vi "HW_GEN - Data Queue Manage FGV.vi"(7 "Oper.":T3=enum."Add", 8 "error in":errorcluster, 10 "ChanTag":string, 11 "Add Chan":T2) -> (0 "error out":errorcluster, 2 "ChanInfo":cluster{"Queue Name":string, "index":i32}, 3 "AllChanInfo":T1(array[cluster]))   [LabVIEW 2016]
uses:
  Ctrls/HardWare _ Data Queue Manage FGV Operation.ctl
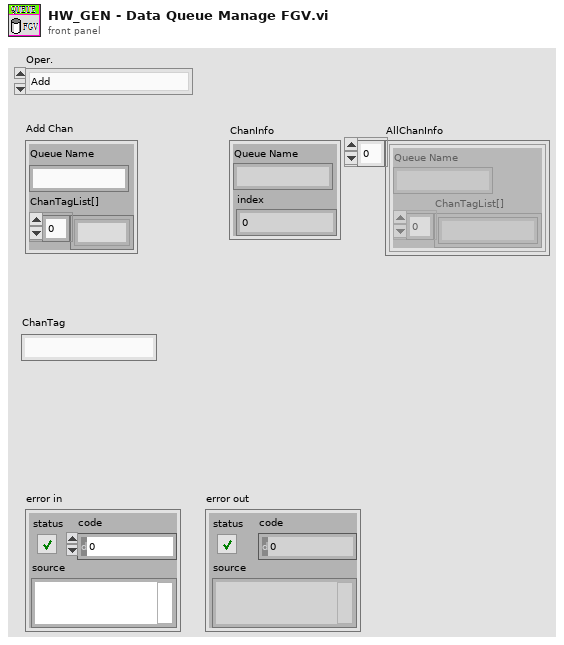
[diagram p1: front panel]
types:
  T1 = cluster{"Queue Name":string, "ChanTagList[]":string[]}[]
  T2 = cluster{"Queue Name":string, "ChanTagList[]":string[]}
  T3 = typedef "HardWare _ Data Queue Manage FGV Operation.ctl" = enum16{"Initialize", "Add", "Read", "All"}
  T4 = cluster{"Queue Name":string, "index of element":i32}
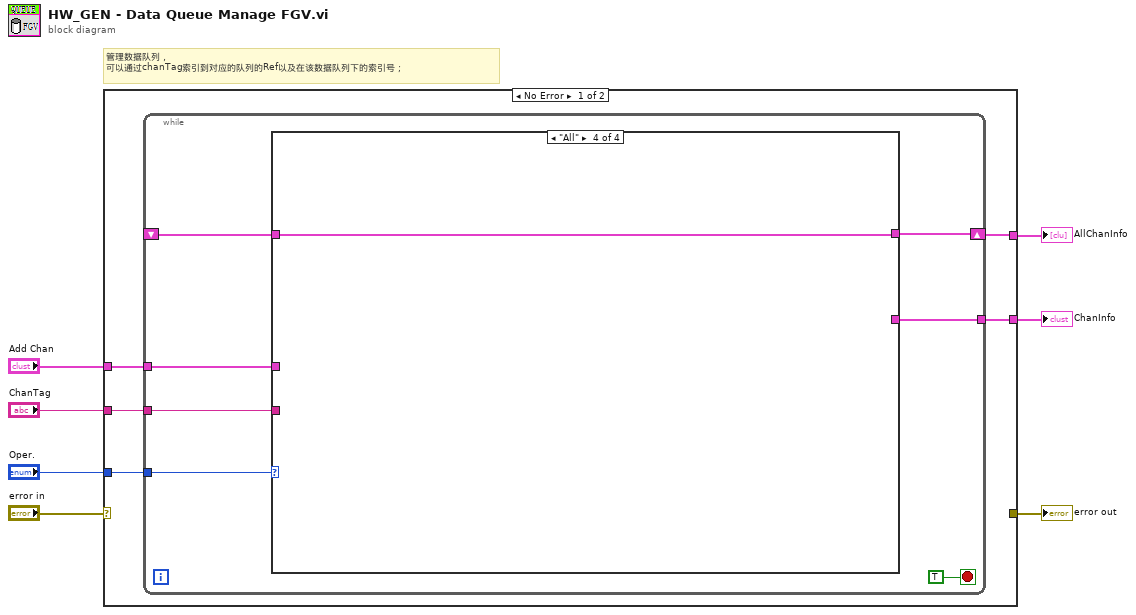
[diagram p0: block diagram]
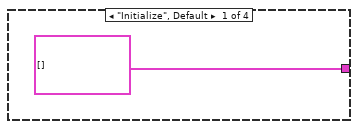
[diagram p2: hidden frame]
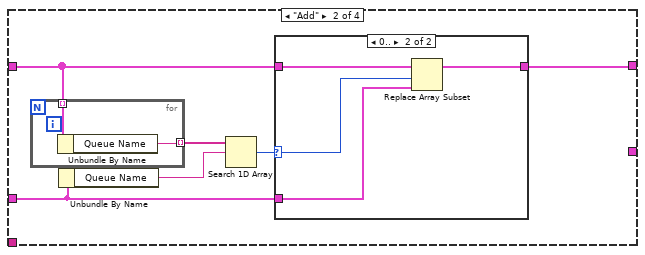
[diagram p3: hidden frame]
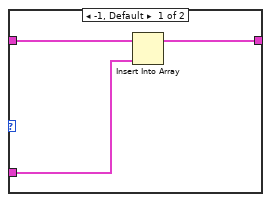
[diagram p4: hidden frame]
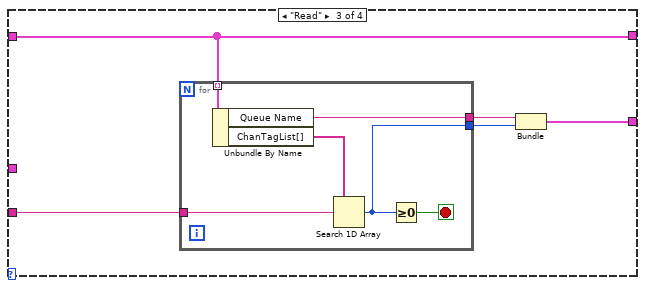
[diagram p5: hidden frame]
diagram:
  # "管理数据队列，\n可以通过chanTag索引到对应的队列的Ref以及在该数据队列下的索引号；"
  n1 = case shown="No Error" "error in" {
    selector: "error in" -> [_ w48]
    tunnel: [_ w48] -> w6
    tunnel: "Oper." -> [w12 _]
    tunnel: "Add Chan" -> [w11 _]
    tunnel: "ChanTag" -> [w10 _]
    tunnel: [w9 _] -> w2
    tunnel: [w8 _] -> w1
    frame No Error {
      n2 = while {
        tunnel: w12 -> [w18]
        tunnel: w11 -> [w17]
        tunnel: w10 -> [w16]
        shift-right: [w15] -> w8
        shift-left: _ -> [w14]
        tunnel: [w13] -> w9
        stop <- TRUE stop-if-true
        n3 = case shown="\"All\"" w18 {
          tunnel: w17 -> [_ w21 _ _]
          tunnel: w16 -> [_ _ w40 _]
          tunnel: [T1 [] w22 w39 w47] -> w15
          tunnel: w14 -> [_ w23 w39 w47]
          tunnel: [_ _ w36 _] -> w13
          frame "Initialize", Default {
          }
          frame "Add" {
            n4 = for {
              tunnel: w23 -> [w35] mode=indexing
              tunnel: [w34] -> w26 mode=indexing
              n5 = Unbundle By Name(w35) -> ("Queue Name"=w34:string)
            }
            n6 = Unbundle By Name(w21) -> ("Queue Name"=w25:string)
            n7 = Search 1D Array(1D array=w26, element=w25) -> (index of element=w24:i32)  [unwired: 1 in]
            n8 = case shown="0.." w24 {
              selector: w24 -> [_ w31]
              tunnel: w23 -> [w29 w33]
              tunnel: [w28 w32] -> w22
              tunnel: w21 -> [w27 w30]
              frame -1, Default {
                n9 = Insert Into Array(array=w29, new element=w27) -> (w28:T1)  [unwired: 1 in]
              }
              frame 0.. {
                n10 = Replace Array Subset(array=w33, new element=w30, index=w31) -> (w32:T1)
              }
            }
          }
          frame "Read" {
            n11 = for {
              tunnel: w39 -> [w46] mode=indexing
              tunnel: w40 -> [w44]
              tunnel: [w42] -> w38
              tunnel: [w41] -> w37
              stop <- w43 stop-if-true
              n12 = Unbundle By Name(w46) -> ("Queue Name"=w42:string, "ChanTagList[]"=w45:string[])
              n13 = Search 1D Array(1D array=w45, element=w44) -> (index of element=w41:i32)  [unwired: 1 in]
              n14 = Greater Or Equal To 0?(x=w41) -> (x >= 0?=w43:bool)
            }
            n15 = Bundle("Queue Name"=w38, "index of element"=w37) -> (w36:T4)  [unwired: 1 in]
          }
          frame "All" {
          }
        }
      }
    }
    frame Error {
    }
  }
  "error out" <- w6
  "ChanInfo" <- w2
  "AllChanInfo" <- w1
